vi "Configure Waveform Characteristics(Phase).vi"(0 "VISA resource name":refnum<visa-resource-name>, 1 "Enable Align (F: Disable)":bool, 5 "Output Channel (1: Channel 1)":i32(ring)=1 items=["Channel 1"=1, "Channel 2"=2], 9 "Phase (0 Degree)":dbl, 11 "error in (no error)":errorcluster) -> (4 "VISA resource name out":refnum<visa-resource-name>, 15 "error out":errorcluster)   [LabVIEW 2012, in "RIGOL DG4000 Series.lvlib"]
doc: "Configures the waveform phase settings."
uses:
  <instrlib>/RIGOL DG4000 Series/RIGOL DG4000 Series.lvlib
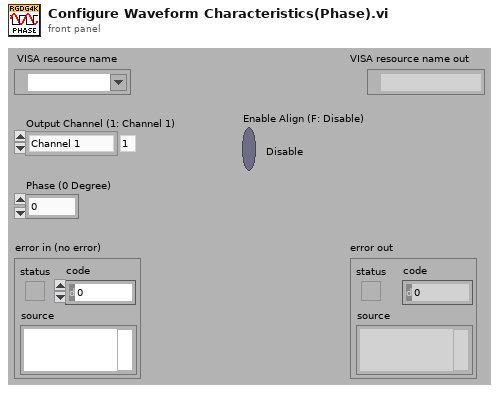
[diagram p1: front panel]
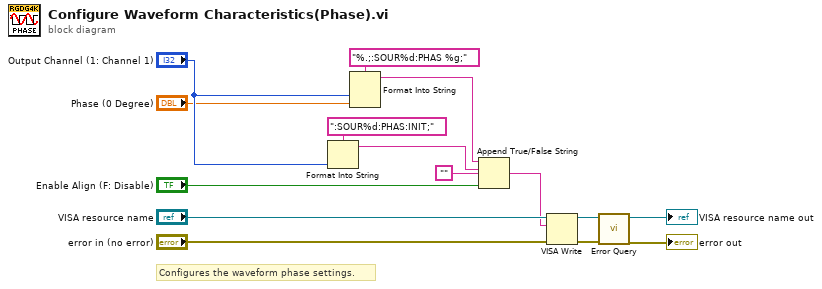
[diagram p0: block diagram]
diagram:
  # "Configures the waveform phase settings."
  n1 = Format Into String(format string=":SOUR%d:PHAS:INIT;", "Output Channel (1: Channel 1)") -> (resulting string=w4:string)  [unwired: 2 in, 1 out]
  n2 = Format Into String(format string="%.;:SOUR%d:PHAS %g;", "Output Channel (1: Channel 1)", "Phase (0 Degree)") -> (resulting string=w5:string)  [unwired: 2 in, 1 out]
  n3 = Append True/False String(1:"Enable Align (F: Disable)", 2:"", 3:w4, 4:w5) -> (0:w1:string)
  n4 = VISA Write(VISA resource name="VISA resource name", write buffer=w1, error in (no error)="error in (no error)") -> (VISA resource name out=w9:refnum<visa-resource-name>, error out=w8:errorcluster)  [unwired: 1 out]
  n5 = call <instrlib>:"Error Query.vi"("error in (no error)"=w8, "VISA resource name"=w9) -> ("error out"=→"error out":errorcluster, "VISA resource name out"=→"VISA resource name out":refnum<visa-resource-name>)  [unwired: 8 out]
